vi "Sort Multi_Run.vi"() -> ()   [LabVIEW 2011]
uses:
  Anemometry Sub Vis/Controls/Tunnel_Coordinates.ctl
  Anemometry Sub Vis/Globals/Trav_pos_global.vi
  Anemometry Sub Vis/Globals/Extra_Commands_Global.vi
panel:
  out "Work in Tunnel Coordinates?":T1
  out "Jump Bad Positions":bool
  in  "Command filename":path
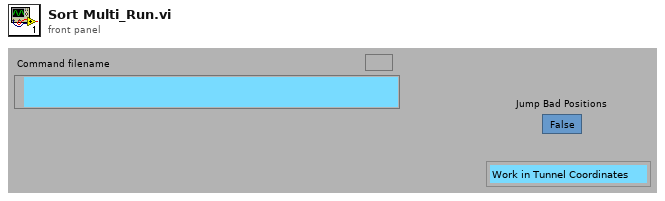
[diagram p1: front panel]
types:
  T1 = typedef "Tunnel_Coordinates.ctl" = enum16{"Work in Tunnel Coordinates", "Work in Model Coordinates"}
  T2 = typedef "Traverse_cluster.ctl" = cluster{"Start X":dbl, "Start Y":dbl, "Start Z":dbl, "End X":dbl, "End Y":dbl, "End Z":dbl, "No. of pts.":i32, "Spacing":T3, "Filename":path, "Tunnel Speed":dbl, "Averaging time (min)":dbl, "Extra Commands":string, "Specific Arguments":string, "Emission Rate (l/min)":dbl, "Trace Gas Concentration (%)":dbl, "Density Ratio":string, "Comments":string, "Row No":i32, "Row Type Selector":T4, "Completion time":string, "Row Duration (mins)":dbl, "No. of Valid pts.":i32, "Meas Setup File":string}
  T3 = typedef "Spacing.ctl" = enum16{"Linear", "Log", "Gauss", "Specified", "N/A"}
  T4 = typedef "Multi_run_mode.ctl" = enum16{"Move Traverse Only", "Set Tunnel Speed Only", "Set Source Only", "Set Measurement Conditions", "Single Measurement", "Vertical Profile", "Lateral Profile", "Longitudinal Profile", "Explore Volume", "Multi-Axis Profile", "Auto Calibrate", "Meas Fast FID Bkgnd", "Check Beam Power", "Scanning Valve Measurement", "Run VI Named:", "Set ADAM Ch", "Wait (minutes)", "Send Message", "Synchronize With:", "Fall Back to this Row", "Turn Off Row Repeating", "Blank Row", "Traverse 3D Volume"}
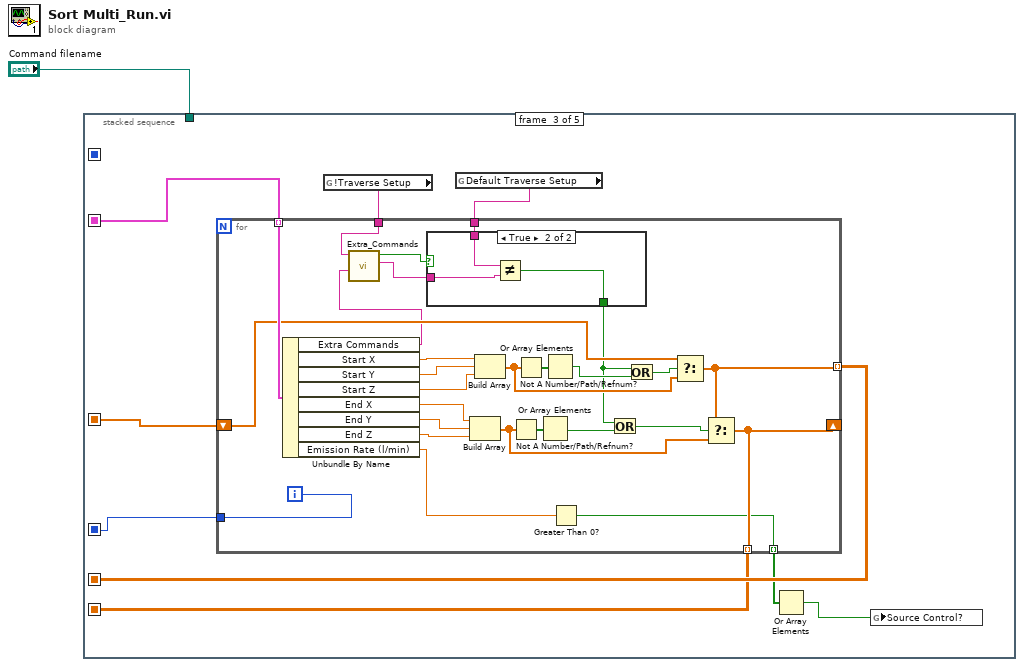
[diagram p0: block diagram]
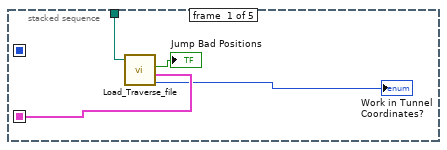
[diagram p2: hidden frame]
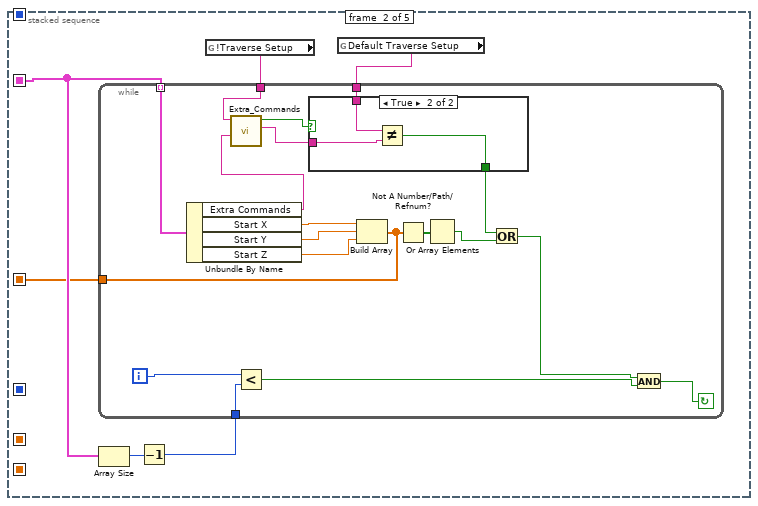
[diagram p3: hidden frame]
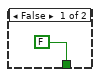
[diagram p4: hidden frame]
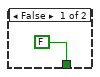
[diagram p5: hidden frame]
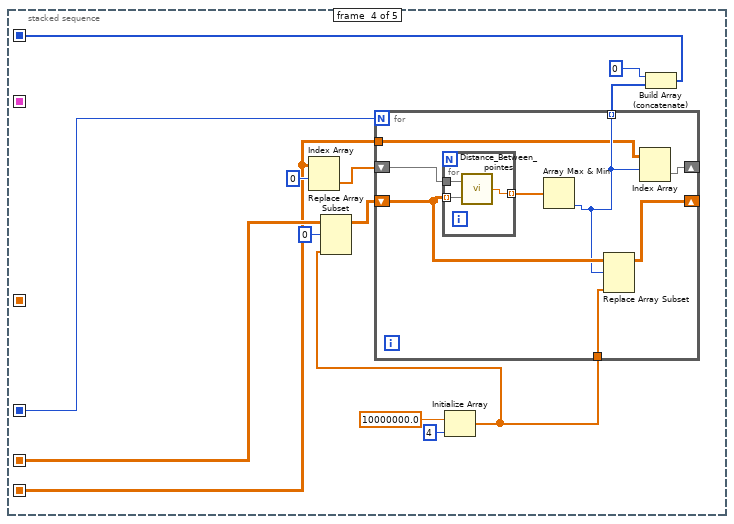
[diagram p6: hidden frame]
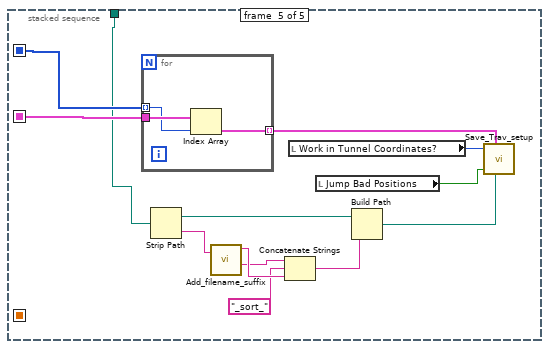
[diagram p7: hidden frame]
diagram:
  n1 = stacked-sequence {
    seq-local: [_ _ w42 _ _] -> [_ _ _ w80 _]
    seq-local: [_ _ w41 _ _] -> [_ _ _ w79 _]
    seq-local: [_ _ w40 _ _] -> [_ _ _ w78 _]
    seq-local: [_ _ _ w75 _] -> [_ _ _ _ w109]
    seq-local: [w4 _ _ _ _] -> [_ w9 w39 _ w110]
    seq-local: [_ w6 _ _ _] -> [_ _ w36 _ _]
    tunnel: "Command filename" -> [w5 _ _ _ w107]
    frame #0 {
      n2 = call "Load_Traverse_file.vi"("Setup filename"=w5) -> ("Jump Bad Positions"=→"Jump Bad Positions":bool, "Table"=w4:T2[], "Work in Tunnel Coordinates?"=→"Work in Tunnel Coordinates?":T1)  [unwired: 3 out]
    }
    frame #1 {
      n3 = Array Size(array=w9) -> (size(s)=w8:i32)
      n4 = Decrement(x=w8) -> (x-1=w7:i32)
      n5 = global read "Extra_Commands_Global.vi" "!Traverse Setup"() -> (w11:string)
      n6 = global read "Trav_pos_global.vi" "Default Traverse Setup"() -> (w10:string)
      n7 = while {
        tunnel: w9 -> [w29] mode=indexing
        tunnel: w11 -> [w24]
        tunnel: w10 -> [w20]
        tunnel: w7 -> [w16]
        tunnel: [w13] -> w6
        i -> [w17]
        stop <- w12 continue-if-true
        n8 = Unbundle By Name(w29) -> ("Extra Commands"=w23:string, "Start X"=w27:dbl, "Start Y"=w26:dbl, "Start Z"=w25:dbl)
        n9 = call "Extra_Commands.vi"("String to Search"=w23, "Command"=w24) -> ("String Value"=w21:string, "Command Found"=w22:bool)  [unwired: 1 in, 3 out]
        n10 = Less?(x=w17, y=w16) -> (x < y?=w15:bool)
        n11 = case shown="True" w22 {
          tunnel: w21 -> [_ w33]
          tunnel: w20 -> [_ w32]
          tunnel: [FALSE w31] -> w18
          frame False {
          }
          frame True {
            n12 = Not Equal?(x=w32, y=w33) -> (x != y?=w31:bool)
          }
        }
        n13 = Build Array(w27, w26, w25) -> (w13:dbl[])
        n14 = Not A Number/Path/Refnum?(number/path/refnum=w13) -> (NaN/Path/Refnum?=w28:bool[])
        n15 = Or Array Elements(Boolean array=w28) -> (logical OR=w19:bool)
        n16 = Or(x=w18, y=w19) -> (x .or. y?=w14:bool)
        n17 = And(x=w14, y=w15) -> (x .and. y?=w12:bool)
      }
    }
    frame #2 {
      n18 = global read "Extra_Commands_Global.vi" "!Traverse Setup"() -> (w38:string)
      n19 = global read "Trav_pos_global.vi" "Default Traverse Setup"() -> (w37:string)
      n20 = for {
        tunnel: w39 -> [w69] mode=indexing
        shift-right: [w56] -> _
        shift-left: w36 -> [w57]
        tunnel: [w58] -> w42 mode=indexing
        tunnel: [w56] -> w41 mode=indexing
        tunnel: [w55] -> w40
        tunnel: w38 -> [w54]
        tunnel: w37 -> [w50]
        tunnel: [w43] -> w34 mode=indexing
        i -> [w55]
        n21 = Unbundle By Name(w69) -> ("Extra Commands"=w53:string, "Start X"=w67:dbl, "Start Y"=w66:dbl, "Start Z"=w65:dbl, "End X"=w61:dbl, "End Y"=w60:dbl, "End Z"=w59:dbl, "Emission Rate (l/min)"=w44:dbl)
        n22 = call "Extra_Commands.vi"("String to Search"=w53, "Command"=w54) -> ("String Value"=w51:string, "Command Found"=w52:bool)  [unwired: 1 in, 3 out]
        n23 = case shown="True" w52 {
          tunnel: w51 -> [_ w73]
          tunnel: w50 -> [_ w72]
          tunnel: [FALSE w71] -> w46
          frame False {
          }
          frame True {
            n24 = Not Equal?(x=w72, y=w73) -> (x != y?=w71:bool)
          }
        }
        n25 = Build Array(w61, w60, w59) -> (w63:dbl[])
        n26 = Build Array(w67, w66, w65) -> (w64:dbl[])
        n27 = Not A Number/Path/Refnum?(number/path/refnum=w63) -> (NaN/Path/Refnum?=w62:bool[])
        n28 = Not A Number/Path/Refnum?(number/path/refnum=w64) -> (NaN/Path/Refnum?=w68:bool[])
        n29 = Or Array Elements(Boolean array=w62) -> (logical OR=w47:bool)
        n30 = Or Array Elements(Boolean array=w68) -> (logical OR=w48:bool)
        n31 = Greater Than 0?(x=w44) -> (x > 0?=w43:bool)
        n32 = Or(x=w46, y=w47) -> (x .or. y?=w45:bool)
        n33 = Or(x=w46, y=w48) -> (x .or. y?=w49:bool)
        n34 = Select(t=w57, s=w49, f=w64) -> (s? t:f=w58:dbl[])
        n35 = Select(t=w58, s=w45, f=w63) -> (s? t:f=w56:dbl[])
      }
      n36 = Or Array Elements(Boolean array=w34) -> (logical OR=w35:bool)
      n37 = global write "Trav_pos_global.vi" "Source Control?"(w35) -> ()
    }
    frame #3 {
      n38 = Index Array(array=w79, index (row)=0) -> (element=w82:dbl[])  [unwired: 1 in]
      n39 = Initialize Array(10000000.0 ("element"), 4 ("dimension size")) -> (w85:dbl[])
      n40 = Replace Array Subset(array=w80, new element=w85, index (row)=0) -> (w86:dbl[][])  [unwired: 1 in]
      n41 = for {
        N: w78 -> [_]
        tunnel: [w89] -> w76 mode=indexing
        shift-right: [w92] -> _
        shift-left: w86 -> [w93]
        shift-right: [w90] -> _
        shift-left: w82 -> [w91]
        tunnel: w79 -> [w88]
        tunnel: w85 -> [w87]
        n42 = for {
          tunnel: w91 -> [w97]
          tunnel: w93 -> [w96] mode=indexing
          tunnel: [w95] -> w94 mode=indexing
          n43 = call "Distance_Between_pointes.vi"("P2"=w96, "P1"=w97) -> ("Distance"=w95:dbl)
        }
        n44 = Array Max & Min(array=w94) -> (min index (indices)=w89:i32)  [unwired: 3 out]
        n45 = Replace Array Subset(array=w93, new element=w87, index (row)=w89) -> (w92:dbl[][])  [unwired: 1 in]
        n46 = Index Array(array=w88, index (row)=w89) -> (element=w90:dbl[])  [unwired: 1 in]
      }
      n47 = Build Array (concatenate)(0 ("min index(es)"), w76) -> (w75:i32[])
    }
    frame #4 {
      n48 = for {
        tunnel: w110 -> [w113]
        tunnel: w109 -> [w112] mode=indexing
        tunnel: [w111] -> w108 mode=indexing
        n49 = Index Array(array=w113, index=w112) -> (element=w111:T2)
      }
      n50 = Strip Path(path=w107) -> (stripped path=w106:path, name=w105:string)
      n51 = call "Add_filename_suffix.vi"("Filename"=w105) -> ("Original Suffix"=w104:string, "Base name"=w98:string)  [unwired: 1 in, 2 out]
      n52 = Concatenate Strings(w98, "_sort_" ("string"), w104) -> (w102:string)
      n53 = local read "Work in Tunnel Coordinates?"() -> (w99:T1)
      n54 = local read "Jump Bad Positions"() -> (w100:bool)
      n55 = Build Path(base path=w106, name or relative path=w102) -> (appended path=w101:path)
      n56 = call "Save_Trav_setup.vi"("Work in Tunnel Coordinates?"=w99, "Trav Table"=w108, "Jump Bad Positions"=w100, "Setup filename"=w101) -> ()  [unwired: 2 out]
    }
  }
